vi "Constructor.vi"(5 "TimeZoneInfoId":string, 6 "MeasureExecutionStatus":T1=enum."NOT_COMPLETED", 7 "MeasureTime":timestamp, 8 "error in":errorcluster, 10 "Value":i64, 11 "Name":string) -> (0 "error out":errorcluster, 3 "IntergerMeasure":refnum<class "IntegerMeasure.lvclass">)   [LabVIEW 2021, in "ProligentXMLGenerator.lvlib" / "IntegerMeasure.lvclass"]
uses:
  IntegerMeasure.lvclass
  IntegerMeasure.lvclass/IntegerMeasure.ctl
  Measure/Measure.lvclass
  Base/MeasureKind/Value.ctl
  Base/MeasureKind/MeasureKind.lvclass
  Data.ctl
  Base/Integer/Integer.lvclass
  C:/Projects/proligent-xml-generator-labview/src/ProligentXMLGenerator/Measure/Measure/Measure.lvclass
  C:/Projects/proligent-xml-generator-labview/src/ProligentXMLGenerator/Measure/IntegerMeasure/IntegerMeasure.lvclass
  Base/ExecutionStatus/Value.ctl
  Base/ExecutionStatus/ExecutionStatus.lvclass
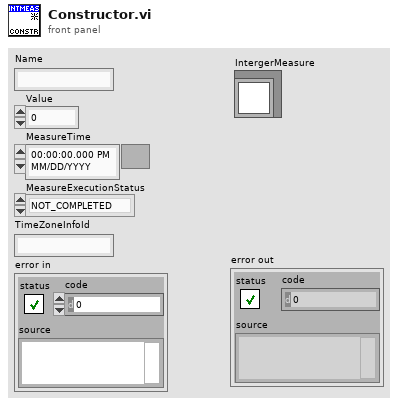
[diagram p1: front panel]
types:
  T1 = typedef "ProligentXMLGenerator.lvlib/ExecutionStatus.lvclass/Value.ctl" = enum16{"PASS", "FAIL", "NOT_COMPLETED", "ABORTED"}
  T2 = typedef "ProligentXMLGenerator.lvlib/IntegerMeasure.lvclass/Data.ctl" = cluster{"Value":refnum<class "Integer.lvclass">}
  T3 = typedef "ProligentXMLGenerator.lvlib/MeasureKind.lvclass/Value.ctl" = enum16{"REAL", "BOOL", "INTEGER", "STRING", "DATETIME"}
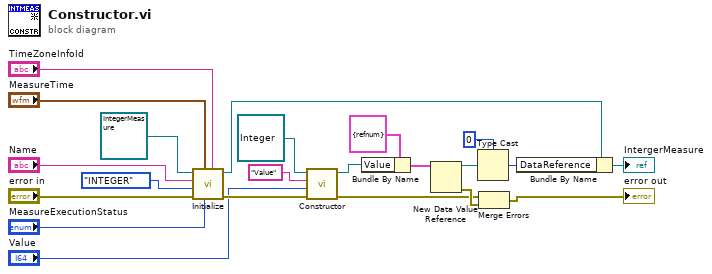
[diagram p0: block diagram]
diagram:
  n1 = call "Initialize.vi"("TimeZoneInfoId"="TimeZoneInfoId", "MeasureExecutionStatus"="MeasureExecutionStatus", "MeasureTime"="MeasureTime", "error in"="error in", "Type"=Value."INTEGER", "Name"="Name", "Measure in"=refnum<class "IntegerMeasure.lvclass"> refnum ("ProligentResultProcessor:RealMeasure")) -> ("error out"=w6:errorcluster, "Measure out"=w17:refnum<class "IntegerMeasure.lvclass">)  [unwired: 3 in]
  n2 = call-dynamic "Constructor.vi"("error in"=w6, "Value"="Value", "Name"="Value", "Integer in"=refnum<class "Integer.lvclass"> refnum ("ProligentResultProcessor:Integer")) -> ("error out"=w2:errorcluster, "Integer out"=w3:refnum<class "Integer.lvclass">)  [unwired: 6 in]
  n3 = Bundle By Name(cluster=T2 {"Value"=refnum} ("Data"), "Value"=w3) -> (w11:T2)
  n4 = New Data Value Reference(data value=w11) -> (data value reference=w18:refnum<data-value>, error out=w21:errorcluster)  [unwired: 1 in]
  n5 = Type Cast(type=u64 0, x=w18) -> (*(type *) &x=w20:u64)
  n6 = Merge Errors(w2, w21) -> (→"error out":errorcluster)
  n7 = Bundle By Name(cluster=w17, "DataReference"=w20) -> (→"IntergerMeasure":refnum<class "IntegerMeasure.lvclass">)
